vi "1_Object_Detection(Train).vi"() -> ()   [LabVIEW 2020]
doc: "This example demonstrates the usage of Deep Learning Toolkit for solving Object Detection problem with Convolutional Neural Network (CNN).\nDataset: Synthetic. Please generate the dataset with \"Dataset_Generation.vi\" in the project.\nRequirements: \n1. Deep Learning Toolkit for LabVIEW.\n2. Vision Development Module."
uses:
  <vilib>/Ngene/Deep Learning Toolkit/Toolkit/NN_Train/Controls/NN_Train_Session_Data.ctl
  <vilib>/Ngene/Deep Learning Toolkit/Toolkit/NN_Train/Controls/NN_LR_Policy_Cfg.ctl
  <vilib>/Ngene/Deep Learning Toolkit/Toolkit/NN_Train/Controls/NN_LR_Policy_Type.ctl
  <vilib>/Ngene/Deep Learning Toolkit/Toolkit/NN_Train/Controls/NN_Train_Params.ctl
  <vilib>/Ngene/Deep Learning Toolkit/Toolkit/NN_Train/Controls/NN_Train_Optimizer.ctl
  <vilib>/Ngene/Deep Learning Toolkit/Toolkit/NN_Train/Controls/NN_Train_Data_Sampling.ctl
  <vilib>/Ngene/Deep Learning Toolkit/Toolkit/NN_Network/Controls/NN_Device.ctl
  <vilib>/Ngene/Deep Learning Toolkit/Toolkit/NN_Loss/API/Controls/NN_Loss_Stats(YOLO_v2).ctl
  <vilib>/Ngene/Deep Learning Toolkit/Toolkit/NN_Data/API/NN_Dims(C,H,W).ctl
  <vilib>/Ngene/Deep Learning Toolkit/Toolkit/NN_Layers/Layers/Input/Controls/NN_Layer_Config(Input3D).ctl
  <vilib>/Ngene/Deep Learning Toolkit/Toolkit/NN_Data/Controls/NN_Data_type.ctl
  <vilib>/Ngene/Deep Learning Toolkit/Toolkit/NN_Network/Controls/NN_Save_Before_Destroy_Options.ctl
  <vilib>/Ngene/Deep Learning Toolkit/Toolkit/NN_Loss/Controls/NN_Loss_Config_Params(YOLO_v4).ctl
  <vilib>/Ngene/Deep Learning Toolkit/Toolkit/NN_Layers/Layers/YOLO_v4/delta_IOU/Controls/IOU_LOSS.ctl
  <vilib>/Ngene/Deep Learning Toolkit/Toolkit/NN_Layers/Layers/Conv2D/Controls/NN_Layer_Config(Conv2D).ctl
  <vilib>/Ngene/Deep Learning Toolkit/Toolkit/NN_Layers/Layers/Conv2D/Controls/NN_Layer_Params(Conv2D).ctl
  <vilib>/Ngene/Deep Learning Toolkit/Toolkit/NN_Layers/Layers/Conv2D/Controls/NN_Conv2D_Padding_Type.ctl
  <vilib>/Ngene/Deep Learning Toolkit/Toolkit/NN_Layers/Layers/BatchNorm/Controls/NN_BN_Params.ctl
  <vilib>/Ngene/Deep Learning Toolkit/Toolkit/NN_Activations/Controls/NN_Activation_Type.ctl
  <vilib>/Ngene/Deep Learning Toolkit/Toolkit/NN_Layers/Controls/NN_Layer_Init_Params.ctl
  <vilib>/Ngene/Deep Learning Toolkit/Toolkit/NN_Layers/Controls/NN_Layer_Weight_Init_Type.ctl
  <vilib>/Ngene/Deep Learning Toolkit/Toolkit/NN_Layers/Layers/YOLO_v4/API/Controls/NN_Layer_Config(YOLO_v4).ctl
  <vilib>/Ngene/Deep Learning Toolkit/Toolkit/NN_Layers/Layers/YOLO_v4/Controls/NN_Layer_Params(YOLO_v4).ctl
  <vilib>/Ngene/Deep Learning Toolkit/Toolkit/NN_Layers/Layers/YOLO_v4/Controls/Box_H_W_Activation_YOLO_v4.ctl
  <vilib>/Ngene/Deep Learning Toolkit/Toolkit/NN_Layers/Layers/DropOut3D/Controls/NN_Layer_Config(DropOut3D).ctl
  94310c40-c364-43de-9d18-57e5de7a2e72.vi
  <vilib>/Ngene/Deep Learning Toolkit/Toolkit/Utils/Vision/Coords_Rect2PolyLine.vi
  <vilib>/Ngene/Deep Learning Toolkit/Toolkit/NN_Layers/Layers/Input/NN_Layer_Create(Input3D).vi
  <vilib>/Ngene/Deep Learning Toolkit/Toolkit/NN_Layers/Layers/Conv2D/NN_Layer_Create(Conv2D).vi
  <vilib>/Ngene/Deep Learning Toolkit/Toolkit/NN_Layers/Layers/DropOut3D/NN_Layer_Create(DropOut3D).vi
  <vilib>/Ngene/Deep Learning Toolkit/Toolkit/NN_Layers/Layers/YOLO_v4/NN_Layer_Create(YOLO_v4).vi
  <vilib>/Ngene/Deep Learning Toolkit/Toolkit/NN_Train/Loss_Functions/NN_Set_Loss(YOLO_v4).vi
  <vilib>/Ngene/Deep Learning Toolkit/Toolkit/NN_Data/subVIs/Dataset/NN_Variant_to_DVR/4D/NN_Data_Variant_to_DVR(4D_SGL).vi
  <vilib>/Ngene/Deep Learning Toolkit/Toolkit/NN_Data/subVIs/Get_Data_Vals/4D/NN_Data_Get_ValByRef(4D_SGL_idx).vi
  <vilib>/Ngene/Deep Learning Toolkit/Toolkit/NN_Network/API/NN_Set_Input/3D/NN_Set_Input(3D_SGL_idx).vi
  <vilib>/Ngene/Deep Learning Toolkit/Toolkit/NN_Network/subVIs/NN_Predict/NN_Predict(In3D_OutBBox).vi
  <vilib>/Ngene/Deep Learning Toolkit/Toolkit/NN_Train/Eval_Loss/NN_Eval_Test_Error_Loss/NN_Eval(In3D_OutBBox).vi
  <vilib>/Ngene/Deep Learning Toolkit/Toolkit/NN_Data/subVIs/Dataset_Destroy/NN_Datasets_All_Destroy(In3D_OutBBox).vi
  <vilib>/Ngene/Deep Learning Toolkit/Toolkit/Deep_Learning_Toolkit_by_Ngene.lvlib
panel:
  in  "Eval Every N Epochs":i32=5
  out "Test.Dataset_Size":i32=74
  out "Train.Dataset_Size":i32=1224
  out "Dims_In":T1={"C"=3, "H"=320, "W"=568}
  in  "Test Dataset (Annotations)":path=path "D:/Ngene/GitHub/deepltk_examples/3_Image_Processing/33_Object_Detection/Dataset/0_Orig/Test/Annotations"
  in  "Test Dataset (Images)":path=path "D:/Ngene/GitHub/deepltk_examples/3_Image_Processing/33_Object_Detection/Dataset/0_Orig/Test/Images"
  in  "Train Dataset (Annotations)":path=path "D:/Ngene/GitHub/deepltk_examples/3_Image_Processing/33_Object_Detection/Dataset/1_Aug(4x)/Train/Annotations"
  out "Train Speed (img/s)":dbl=167.44125689875221 format="%#_2p"
  out "Session Data":T2={"Epochs"=18.130718, "Tot_Iter"=1387, "LR"=0.005, "LR_iter"=1388}
  in  "Stop":bool
  in  "LR Update Policy":T3={"Policy_Type"=enum."Step", "LR0"=0.01, "k"=15.0, "WarmUp_Policy"=enum."Ramp", "WarmUp_Iter"=1000, "WarmUp_Ratio"=10.0} {"WarmUp_Ratio" min=1; "WarmUp_Iter" min=1; "LR0" format="%.7f"}
  out "Train Speed (s/iter)":dbl=0.09555589999945369 format="%#_2p"
  in  "Train_Params":T5={"Optimizer"=enum."Adam", "Beta_1"=0.9, "Beta_2"=0.999, "Weight Decay(L1)"=4e-07, "Weight Decay(L2)"=4e-07, "Data_Sampling"=enum."Random"}
  out "Time_Elapsed":dbl=141.26338669999677 format="%<%H:%M:%S>t"
  in  "Working Dir":path=path "D:/working"
  in  "NN_Device":T8=enum."GPU"
  in  "Train Dataset (Images)":path=path "D:/Ngene/GitHub/deepltk_examples/3_Image_Processing/33_Object_Detection/Dataset/1_Aug(4x)/Train/Images"
  out "Loss_Stats":T9={"Avg_Recall"=0.994248, "Avg_Class"=0.99027264, "Avg_Obj"=0.814741, "Avg_IOU"=0.83733565, "Avg_NoObj"=0.014255692, "Count"=267, "Loss"=6.247297} {"Loss" format="%.5f"; "Count" format="%.5f"; "Avg_NoObj" format="%.5f"; "Avg_IOU" format="%.5f"; "Avg_Obj" format="%.5f"; "Avg_Class" format="%.5f"; "Avg_Recall" format="%.5f"}
  out "Loss_Stats_Graph":T10(graph)={"Avg_recall"=0.994248, "Avg_cat"=0.814741, "Avg_obj"=0.83733565, "Avg_iou"=0.014255692, "Avg_NoObj"=6.247297, "Count"=0.80606145, "Loss"=0.98615247}
  out "Prediction":T11(plugin-control)
  in  "IOU_Thresh(NMS)":sgl=0.42
  in  "Confidence_Thresh":sgl=0.49999997
  in  "Display?":bool
  in  "Evaluate":bool
  out "Mean_IoU":sgl=0.80606145 format="%#_4g"
  out "mAP":sgl=0.98615247 format="%#_4g"
  in  "Select Sample":i32=14 min=0 max=73 step=1
  # "4. In order to be able to observe detection results on a specific sample in a dataset set \"Display?\" to True and select sample with help of \"Select Sample\" control.\n7. Change the \"Confidence_Threshold\" and  \"IOU_Thresh(NMS)\" to observe their influence on detection results.\n8. Unselect \"Display\" button to speed up the training.\n10. Press \"Evaluate\" to measure network performance on Test dataset..\n11.  Stop the training when Loss is not decreasing any more.\n12. (Optional) Change \"NN_Device\" value to \"GPU\" to compare execution speeds on GPU and CPU.\n\nMore Examples:  https://github.com/ngenehub/deepltk_examples"
  # "Overview: This example demonstrates the usage of Deep Learning Toolkit for solving Object Detection problem with Convolutional Neural Network (YOLO v4).\nRequirements: \n1. Deep Learning Toolkit for LabVIEW.\n2. Vision Development Module.\nInstructions:\n1. Provide paths to Training and Test datasets at \"Train Dataset (Images)\", \"Train Dataset (Annotations)\", \"Test Dataset (Images)\", and \"Test Dataset (Annotations)\". \n2. Set appropriate path at \"Working Dir\" control where the results of the training will be stored.\n3. Run the VI with current configuration of parameters and observe the training process."
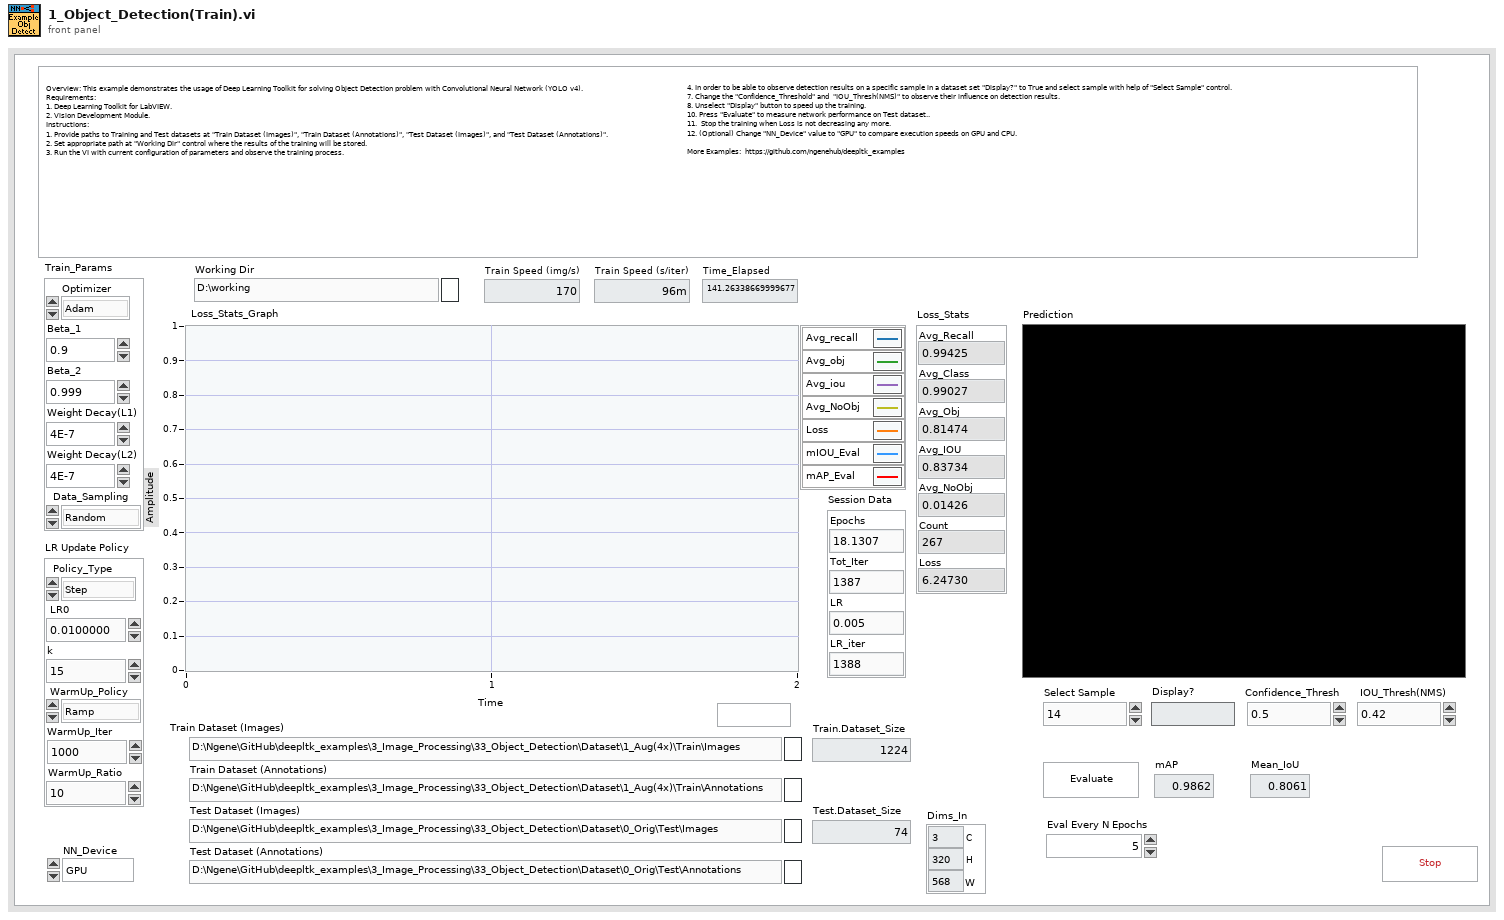
[diagram p1: front panel]
types:
  T1 = typedef "Deep_Learning_Toolkit_by_Ngene.lvlib/NN_Dims(C,H,W).ctl" = cluster{"C":i32, "H":i32, "W":i32}
  T2 = typedef "Deep_Learning_Toolkit_by_Ngene.lvlib/NN_Train_Session_Data.ctl" = cluster{"Epochs":sgl, "Tot_Iter":i32, "LR":sgl, "LR_iter":i32}
  T3 = typedef "Deep_Learning_Toolkit_by_Ngene.lvlib/NN_LR_Policy_Cfg.ctl" = cluster{"Policy_Type":T4, "LR0":dbl, "k":sgl, "WarmUp_Policy":enum16{"Step", "Ramp"}, "WarmUp_Iter":i32, "WarmUp_Ratio":sgl}
  T4 = typedef "Deep_Learning_Toolkit_by_Ngene.lvlib/NN_LR_Policy_Type.ctl" = enum16{"Manual", "Step", "Exp", "1/t"}
  T5 = typedef "Deep_Learning_Toolkit_by_Ngene.lvlib/NN_Train_Params.ctl" = cluster{"Optimizer":T6, "Beta_1":sgl, "Beta_2":sgl, "Weight Decay(L1)":sgl, "Weight Decay(L2)":sgl, "Data_Sampling":T7}
  T6 = typedef "Deep_Learning_Toolkit_by_Ngene.lvlib/NN_Train_Optimizer.ctl" = enum16{"SGD", "Adam", "Adagrad", "Adadelta", "RMSProp", "Nesterov"}
  T7 = typedef "Deep_Learning_Toolkit_by_Ngene.lvlib/NN_Train_Data_Sampling.ctl" = enum16{"Random", "Sequential"}
  T8 = typedef "Deep_Learning_Toolkit_by_Ngene.lvlib/NN_Device.ctl" = enum16{"CPU", "GPU"}
  T9 = typedef "Deep_Learning_Toolkit_by_Ngene.lvlib/NN_Loss_Stats(YOLO_v2).ctl" = cluster{"Avg_Recall":sgl, "Avg_Class":sgl, "Avg_Obj":sgl, "Avg_IOU":sgl, "Avg_NoObj":sgl, "Count":i32, "Loss":sgl}
  T10 = cluster{"Avg_recall":sgl, "Avg_cat":sgl, "Avg_obj":sgl, "Avg_iou":sgl, "Avg_NoObj":sgl, "Count":sgl, "Loss":sgl}
  T11 = typedef "IMAQ Image.ctl" = refnum<image>
  T12 = typedef "Deep_Learning_Toolkit_by_Ngene.lvlib/NN_Layer_Config(DropOut3D).ctl" = cluster{"Name":string, "Probability":sgl}
  T13 = typedef "Deep_Learning_Toolkit_by_Ngene.lvlib/NN_Layer_Config(YOLO_v4).ctl" = cluster{"Name":string, "YOLO_v4_Params":T14, "Custom_Params":string}
  T14 = typedef "Deep_Learning_Toolkit_by_Ngene.lvlib/NN_Layer_Params(YOLO_v4).ctl" = cluster{"classes":i32, "anchors":sgl[][], "Box_H_W_Activation":T15, "Box_H_W_Scale":sgl, "Box_X_Y_Scale":sgl}
  T15 = typedef "Deep_Learning_Toolkit_by_Ngene.lvlib/Box_H_W_Activation_YOLO_v4.ctl" = enum16{"Exponent", "Sigmoid"}
  T16 = typedef "Deep_Learning_Toolkit_by_Ngene.lvlib/NN_Layer_Config(Conv2D).ctl" = cluster{"Name":string, "Conv_Params":T17, "BN?":bool, "BN_Params":T19, "Activation":T20, "Has Bias?":bool, "Init_Params":T21, "Custom_Params":string}
  T17 = typedef "Deep_Learning_Toolkit_by_Ngene.lvlib/NN_Layer_Params(Conv2D).ctl" = cluster{"Filters":i32, "Kernel_Size":i32, "Stride":i32, "Pad_Type":T18, "Pad_Size":i32}
  T18 = typedef "Deep_Learning_Toolkit_by_Ngene.lvlib/NN_Conv2D_Padding_Type.ctl" = enum16{"Pad_Size", "Valid", "Same"}
  T19 = typedef "Deep_Learning_Toolkit_by_Ngene.lvlib/NN_BN_Params.ctl" = cluster{"epsilon":sgl, "momentum":sgl}
  T20 = typedef "Deep_Learning_Toolkit_by_Ngene.lvlib/NN_Activation_Type.ctl" = enum16{"Sigmoid", "ReLU", "LReLU", "ReLU6", "tanh", "Swish", "Mish", "None"}
  T21 = typedef "Deep_Learning_Toolkit_by_Ngene.lvlib/NN_Layer_Init_Params.ctl" = cluster{"Init_Type":T22, "Value":sgl}
  T22 = typedef "Deep_Learning_Toolkit_by_Ngene.lvlib/NN_Layer_Weight_Init_Type.ctl" = enum16{"Const", "Uniform", "Gaussian", "Xavier"}
  T23 = typedef "Deep_Learning_Toolkit_by_Ngene.lvlib/NN_Loss_Config_Params(YOLO_v4).ctl" = cluster{"noobject_conf_thresh ":sgl, "object_scale":sgl, "class_scale":sgl, "coord_scale":sgl, "noobject_scale":sgl, "obj_to_IOU_power":sgl, "IOU_loss":T24}
  T24 = typedef "Deep_Learning_Toolkit_by_Ngene.lvlib/IOU_LOSS.ctl" = enum16{"MSE", "IOU", "GIOU", "DIOU", "CIOU"}
  T25 = typedef "Image Type" = u32
  T26 = typedef "Deep_Learning_Toolkit_by_Ngene.lvlib/NN_Save_Before_Destroy_Options.ctl" = cluster{"CFG?":bool, "Weights?":bool, "Render?":bool}
  T27 = typedef "Deep_Learning_Toolkit_by_Ngene.lvlib/NN_Layer_Config(Input3D).ctl" = cluster{"Name":string, "Dims":T1, "Data_Type":T28, "Shifts":sgl[], "Scales":sgl[]}
  T28 = typedef "Deep_Learning_Toolkit_by_Ngene.lvlib/NN_Data_type.ctl" = enum16{"I8", "U8", "I16", "U16", "U32 ARGB", "SGL"}
  T29 = typedef "Deep_Learning_Toolkit_by_Ngene.lvlib/NN_DataSets_All(In3D_OutBBox).ctl" = cluster{"Train":T30, "Validation":T30, "Test":T30}
  T30 = typedef "Deep_Learning_Toolkit_by_Ngene.lvlib/NN_DataSet(In3D_OutBBox).ctl" = cluster{"Inputs Ref.":variant, "Dataset_Size":i32, "Dims_In":T1, "Outputs Refs":T31, "No of Classes ":i32, "Labels":string[], "File Paths":path[]}
  T31 = typedef "Deep_Learning_Toolkit_by_Ngene.lvlib/NN_Data_ref(1D_BBox).ctl" = refnum<data-value>
  T32 = typedef "Deep_Learning_Toolkit_by_Ngene.lvlib/NN.ctl" = cluster{"Name":string, "No of Layers":i32, "mBatch":i32, "Layers":T33[], "Dimty":T34, "Dims_In":T1, "Dims_Out":T1, "Working_Dir":path, "Train?":bool, "Train_Params":T5, "LR_Update_Policy":T3, "Session Data":T2, "Ground_truth":T35, "NNg_hdls":T36, "NN_Device":T8, "GPU Id":i32, "Labels":string[], "Receptive Field":T37[], "Loss_Type":T38, "Loss_Cfg_Prms":variant, "NNG_WS":T39}
  T33 = typedef "Deep_Learning_Toolkit_by_Ngene.lvlib/NN_Layer_ref.ctl" = refnum<data-value>
  T34 = typedef "Deep_Learning_Toolkit_by_Ngene.lvlib/NN_In_Out_Dim-ty.ctl" = enum8{"In1D_Out1D", "In3D_Out1D", "In3D_Out3D", "In3D_OutBBox"}
  T35 = typedef "Deep_Learning_Toolkit_by_Ngene.lvlib/NN_Ground_truth.ctl" = cluster{"Y":variant}
  T36 = typedef "Deep_Learning_Toolkit_by_Ngene.lvlib/nng_cuda_handles.ctl" = cluster{"cudnn":u64, "cublas":u64, "stream":u64, "curand":u64}
  T37 = typedef "Deep_Learning_Toolkit_by_Ngene.lvlib/NN_Dims(V,H).ctl" = cluster{"V":i32, "H":i32}
  T38 = typedef "Deep_Learning_Toolkit_by_Ngene.lvlib/NN_Loss_Type.ctl" = enum16{"None", "MSE", "CrossEntropy", "YOLO_v2", "YOLO_v4"}
  T39 = typedef "Deep_Learning_Toolkit_by_Ngene.lvlib/NNG_WS.ctl" = cluster{"NNG_WS_Mem":T40, "Max_WS_Size":i64}
  T40 = typedef "Deep_Learning_Toolkit_by_Ngene.lvlib/NNg_WS_Mem_DVR.ctl" = refnum<data-value>
  T41 = typedef "Deep_Learning_Toolkit_by_Ngene.lvlib/NN_Data_ref(4D_SGL).ctl" = refnum<data-value>
  T42 = typedef "Deep_Learning_Toolkit_by_Ngene.lvlib/NN_Layer.ctl" = cluster{"Name":string, "Layer_Data":variant, "Layer_Type":T43, "Dims_In":T1, "Layers_In":variant, "Dims_Out":T1, "Layers_Out":variant, "Metrics":T44, "GPU_Data":variant, "mBatch":i32, "NN_Device":T8, "NNg_hdls":T36, "Train?":bool, "Dimty":T45, "RecptField":T46}
  T43 = typedef "Deep_Learning_Toolkit_by_Ngene.lvlib/NN_Layer_Type.ctl" = enum16{"Input1D", "Input3D", "Conv1D", "Conv2D", "Conv2D_Adv", "MaxPool", "AvgPool", "UpSample", "DropOut3D", "ShortCut", "Concat", "SoftMax3D", "FC", "DropOut", "Softmax", "Flatten", "YOLO_v2", "YOLO_v4", "Activation", "BatchNormalization", "Unsupported"}
  T44 = typedef "Deep_Learning_Toolkit_by_Ngene.lvlib/NN_Layer_Metrics.ctl" = cluster{"Data":dbl, "Params":dbl, "Ops":dbl}
  T45 = typedef "Deep_Learning_Toolkit_by_Ngene.lvlib/NN_Layer_Dimty.ctl" = enum16{"1D", "3D"}
  T46 = typedef "Deep_Learning_Toolkit_by_Ngene.lvlib/NN_Layer_RF_State.ctl" = cluster{"Dims":T37, "J":T37}
  T47 = typedef "Deep_Learning_Toolkit_by_Ngene.lvlib/NN_BBox_Detection.ctl" = cluster{"Class":i32, "Conf Level":sgl, "BBox":T48}
  T48 = typedef "Deep_Learning_Toolkit_by_Ngene.lvlib/NN_BBox.ctl" = cluster{"x":sgl, "y":sgl, "w":sgl, "h":sgl}
  T49 = cluster{"Avg_recall":sgl, "Avg_obj":sgl, "Avg_iou":sgl, "Avg_NoObj":sgl, "Loss":sgl, "Mean_IoU":sgl, "mAP":sgl}
  T50 = typedef "Deep_Learning_Toolkit_by_Ngene.lvlib/NN_Image_Detections.ctl" = cluster{"Image Detections":T47[]}
  T51 = typedef "Deep_Learning_Toolkit_by_Ngene.lvlib/NN_Eval_Params(in3D_OutBBox).ctl" = cluster{"Precision@Max_Avg_F1_Score":sgl, "Recall@Max_Avg_F1_Score":sgl, "argmax_avgF1_Score(Conf)":sgl, "Max_Avg_F1_Score":sgl, "Max_F1_Score_Per_Class":sgl[], "F1_Score_Per_Class":sgl[][], "Avg_F1,P,R Curves":cluster{"Conf":sgl[], "F1|P|R":sgl[]}[], "mIOU":sgl, "APs@0.5":sgl[], "PR_Curves@0.5":T52, "IOUs":sgl[], "mAP@0.75":sgl, "mAP@0.5-0.95":sgl, "mAP@0.5":sgl, "Mean_PR_Curve":T53}
  T52 = typedef "Deep_Learning_Toolkit_by_Ngene.lvlib/NN_PR_Curves.ctl" = T53[]
  T53 = typedef "Deep_Learning_Toolkit_by_Ngene.lvlib/NN_PR.ctl" = cluster{"Recall":sgl[], "Precision":sgl[]}
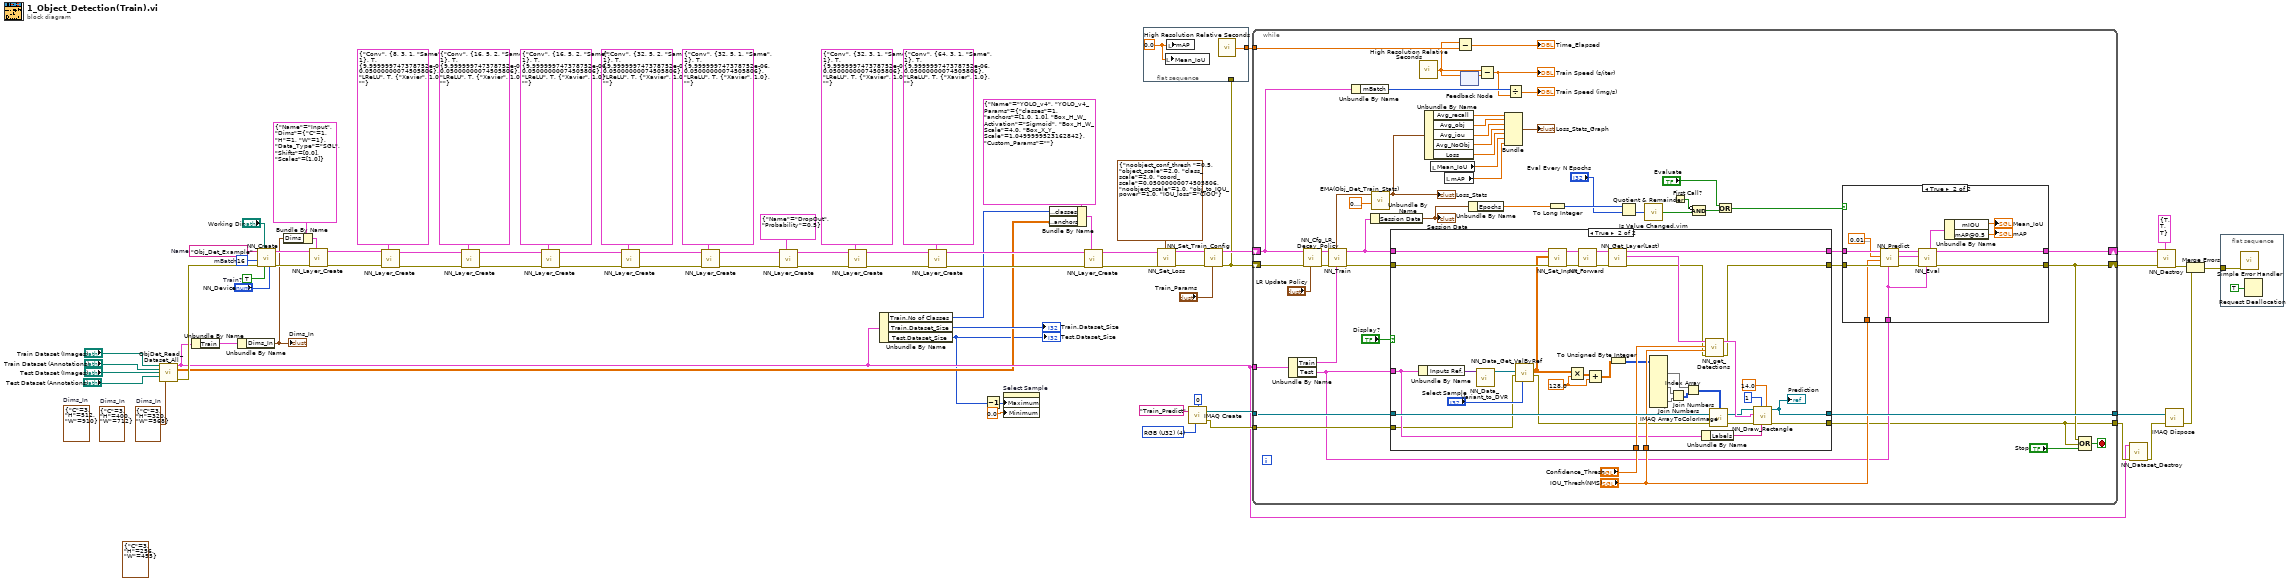
[diagram p0: block diagram]
diagram:
  (unwired) T1 {"C"=3, "H"=400, "W"=712}  # Dims_In
  w1 = T1 {"C"=3, "H"=320, "W"=568}  # Dims_In
  (unwired) T1 {"C"=3, "H"=256, "W"=455} ("Dims(C,H,W)")
  (unwired) T1 {"C"=3, "H"=512, "W"=910}  # Dims_In
  w52 = T25 4 items=["Grayscale (U8)", "Grayscale (I16)", "Grayscale (SGL)", "Complex (CSG)", "RGB (U32)", "HSL (U32)", "RGB (U64)", "Grayscale (U16)"] ("Image Type")
  w61 = TRUE  # Train?
  w67 = 16  # mBatch
  w74 = "Obj_Det_Example"  # Name
  n1 = call "ObjDet_Read_Dataset_All.vi"("Train Image Path"="Train Dataset (Images)", "Train Anno Path"="Train Dataset (Annotations)", "Test Image Path"="Test Dataset (Images)", "Test Anno Path"="Test Dataset (Annotations)", "Dims(C,H,W)"=w1) -> ("Dataset"=w33:T29, "Anchors"=w30:dbl[][], "error out"=w75:errorcluster)  [unwired: 8 in]
  n2 = Unbundle By Name(w33) -> ("Train"=w40:T30)
  n3 = Unbundle By Name(w40) -> ("Dims_In"=w34:T1)
  "Dims_In" <- w34
  n4 = call <vilib>:"NN_Create.vi"("NN_Device"="NN_Device", "Train? (false)"=w61, "Working Dir"="Working Dir", "error in (no error)"=w75, "mBatch (1)"=w67, "Name"=w74) -> ("error out"=w72:errorcluster, "NN out"=w73:T32)  [unwired: 4 in]
  n5 = Bundle By Name(cluster=T27 {"Name"="Input", "Dims"={"C"=1, "H"=1, "W"=1}, "Data_Type"=enum."SGL", "Shifts"=[0.0], "Scales"=[1.0]} ("Cluster"), "Dims"=w34) -> (w37:T27)
  n6 = call-poly <vilib>:"NN_Layer_Create.vi"("Input3D_Cfg"=w37, "error in (no error)"=w72, "NN In"=w73) -> ("error out"=w58:errorcluster, "NN out"=w41:T32)  [unwired: 6 in, 1 out]
  n7 = call-poly <vilib>:"NN_Layer_Create.vi"("Conv2D_Cfg"=T16 {"Name"="Conv", "Conv_Params"={"Filters"=8, "Kernel_Size"=3, "Stride"=1, "Pad_Type"=enum."Same", "Pad_Size"=1}, "BN?"=TRUE, "BN_Params"={"epsilon"=1e-05, "momentum"=0.05}, "Activation"=enum."LReLU", "Has Bias?"=TRUE, "Init_Params"={"Init_Type"=enum."Xavier", "Value"=1.0}, "Custom_Params"=""} ("Layer_Config_Params"), "error in (no error)"=w58, "NN in"=w41) -> ("error out"=w13:errorcluster, "NN out"=w14:T32)  [unwired: 6 in, 1 out]
  n8 = call-poly <vilib>:"NN_Layer_Create.vi"("Conv2D_Cfg"=T16 {"Name"="Conv", "Conv_Params"={"Filters"=16, "Kernel_Size"=5, "Stride"=2, "Pad_Type"=enum."Same", "Pad_Size"=1}, "BN?"=TRUE, "BN_Params"={"epsilon"=1e-05, "momentum"=0.05}, "Activation"=enum."LReLU", "Has Bias?"=TRUE, "Init_Params"={"Init_Type"=enum."Xavier", "Value"=1.0}, "Custom_Params"=""} ("Layer_Config_Params"), "error in (no error)"=w13, "NN in"=w14) -> ("error out"=w21:errorcluster, "NN out"=w22:T32)  [unwired: 6 in, 1 out]
  n9 = call-poly <vilib>:"NN_Layer_Create.vi"("Conv2D_Cfg"=T16 {"Name"="Conv", "Conv_Params"={"Filters"=16, "Kernel_Size"=5, "Stride"=2, "Pad_Type"=enum."Same", "Pad_Size"=1}, "BN?"=TRUE, "BN_Params"={"epsilon"=1e-05, "momentum"=0.05}, "Activation"=enum."LReLU", "Has Bias?"=TRUE, "Init_Params"={"Init_Type"=enum."Xavier", "Value"=1.0}, "Custom_Params"=""} ("Layer_Config_Params"), "error in (no error)"=w21, "NN in"=w22) -> ("error out"=w17:errorcluster, "NN out"=w18:T32)  [unwired: 6 in, 1 out]
  n10 = call-poly <vilib>:"NN_Layer_Create.vi"("Conv2D_Cfg"=T16 {"Name"="Conv", "Conv_Params"={"Filters"=32, "Kernel_Size"=5, "Stride"=2, "Pad_Type"=enum."Same", "Pad_Size"=1}, "BN?"=TRUE, "BN_Params"={"epsilon"=1e-05, "momentum"=0.05}, "Activation"=enum."LReLU", "Has Bias?"=TRUE, "Init_Params"={"Init_Type"=enum."Xavier", "Value"=1.0}, "Custom_Params"=""} ("Layer_Config_Params"), "error in (no error)"=w17, "NN in"=w18) -> ("error out"=w11:errorcluster, "NN out"=w12:T32)  [unwired: 6 in, 1 out]
  n11 = call-poly <vilib>:"NN_Layer_Create.vi"("Conv2D_Cfg"=T16 {"Name"="Conv", "Conv_Params"={"Filters"=32, "Kernel_Size"=5, "Stride"=1, "Pad_Type"=enum."Same", "Pad_Size"=1}, "BN?"=TRUE, "BN_Params"={"epsilon"=1e-05, "momentum"=0.05}, "Activation"=enum."LReLU", "Has Bias?"=TRUE, "Init_Params"={"Init_Type"=enum."Xavier", "Value"=1.0}, "Custom_Params"=""} ("Layer_Config_Params"), "error in (no error)"=w11, "NN in"=w12) -> ("error out"=w16:errorcluster, "NN out"=w4:T32)  [unwired: 6 in, 1 out]
  n12 = call-poly <vilib>:"NN_Layer_Create.vi"("DropOut3D_Cfg"=T12 {"Name"="DropOut", "Probability"=0.5}, "error in (no error)"=w16, "NN in"=w4) -> ("error out"=w5:errorcluster, "NN out"=w3:T32)  [unwired: 6 in, 1 out]
  n13 = call-poly <vilib>:"NN_Layer_Create.vi"("Conv2D_Cfg"=T16 {"Name"="Conv", "Conv_Params"={"Filters"=32, "Kernel_Size"=3, "Stride"=1, "Pad_Type"=enum."Same", "Pad_Size"=1}, "BN?"=TRUE, "BN_Params"={"epsilon"=1e-05, "momentum"=0.05}, "Activation"=enum."LReLU", "Has Bias?"=TRUE, "Init_Params"={"Init_Type"=enum."Xavier", "Value"=1.0}, "Custom_Params"=""} ("Layer_Config_Params"), "error in (no error)"=w5, "NN in"=w3) -> ("error out"=w24:errorcluster, "NN out"=w25:T32)  [unwired: 6 in, 1 out]
  n14 = Unbundle By Name(w33) -> ("Train.No of Classes"=w31:i32, "Train.Dataset_Size"=→"Train.Dataset_Size":i32, "Test.Dataset_Size"=w6:i32)
  "Test.Dataset_Size" <- w6
  n15 = call-poly <vilib>:"NN_Layer_Create.vi"("Conv2D_Cfg"=T16 {"Name"="Conv", "Conv_Params"={"Filters"=64, "Kernel_Size"=3, "Stride"=1, "Pad_Type"=enum."Same", "Pad_Size"=1}, "BN?"=TRUE, "BN_Params"={"epsilon"=1e-05, "momentum"=0.05}, "Activation"=enum."LReLU", "Has Bias?"=TRUE, "Init_Params"={"Init_Type"=enum."Xavier", "Value"=1.0}, "Custom_Params"=""} ("Layer_Config_Params"), "error in (no error)"=w24, "NN in"=w25) -> ("error out"=w38:errorcluster, "NN out"=w39:T32)  [unwired: 6 in, 1 out]
  n16 = Decrement(x=w6) -> (x-1=w8:i32)
  n17 = property on="Select Sample" class="DigNum (strict)"("Maximum"=w8, "Minimum"=0.0 ("Data Entry Limits:Minimum")) -> ()  [unwired: 2 in, 2 out]
  n18 = Bundle By Name(cluster=T13 {"Name"="YOLO_v4", "YOLO_v4_Params"={"classes"=1, "anchors"=[[1.0, 1.0]], "Box_H_W_Activation"=enum."Sigmoid", "Box_H_W_Scale"=4.0, "Box_X_Y_Scale"=1.05}, "Custom_Params"=""} ("YOLO_v4_Cfg"), "YOLO_v4_Params.classes"=w31, "YOLO_v4_Params.anchors"=w30) -> (w9:T13)
  n19 = call-poly <vilib>:"NN_Layer_Create.vi"("YOLO_v4_Cfg"=w9, "error in (no error)"=w38, "NN in"=w39) -> ("error out"=w53:errorcluster, "NN out"=w65:T32)  [unwired: 6 in, 1 out]
  n20 = flat-sequence {
    tunnel: [w77] -> w69
    tunnel: w62 -> [_]
    frame #0 {
      w76 = sgl 0.0 ("mAP")
      n21 = local write "Mean_IoU"(w76) -> ()
      n22 = local write "mAP"(w76) -> ()
      n23 = call <vilib>:"High Resolution Relative Seconds.vi"() -> ("relative seconds"=w77:dbl)
    }
  }
  n24 = call-poly <vilib>:"NN_Set_Loss.vi"("Loss_Config_Params(YOLO_v4)"=T23 {"noobject_conf_thresh "=0.5, "object_scale"=2.0, "class_scale"=2.0, "coord_scale"=0.05, "noobject_scale"=1.0, "obj_to_IOU_power"=1.0, "IOU_loss"=enum."CIOU"}, "error in (no error)"=w53, "NN in"=w65) -> ("error out"=w56:errorcluster, "NN out"=w57:T32)  [unwired: 7 in]
  n25 = call "IMAQ Create"("Border Size"=0, "Image Name"="Train_Predict", "Image Type"=w52) -> ("New Image"=w49:T11, "error out"=w48:errorcluster)  [unwired: 2 in]
  n26 = call <vilib>:"NN_Set_Train_Config.vi"("NN_Train_Params"="Train_Params", "error in (no error)"=w56, "NN in"=w57) -> ("error out"=w62:errorcluster, "NN out"=w63:T32)  [unwired: 7 in]
  n27 = while {
    shift-right: [w105] -> w66
    shift-left: w62 -> [w114]
    shift-right: [w79] -> w70
    shift-left: w63 -> [w115]
    tunnel: w69 -> [w123]
    tunnel: w49 -> [w111]
    tunnel: [w110] -> w47
    tunnel: w48 -> [w109]
    tunnel: [w78] -> w45
    tunnel: w33 -> [w101]
    stop <- w126 stop-if-true
    n28 = Unbundle By Name(w101) -> ("Train"=w99:T30, "Test"=w98:T30)
    n29 = call <vilib>:"NN_Cfg_LR_Decay_Policy.vi"("LR_Decay_Params"="LR Update Policy", "error in (no error)"=w114, "NN in"=w115) -> ("error out"=w124:errorcluster, "NN out"=w127:T32)  [unwired: 7 in]
    n30 = call <vilib>:"NN_Train.vi"("Train Dataset"=w99, "error in (no error)"=w124, "NN in"=w127) -> ("error out"=w112:errorcluster, "NN out"=w113:T32, "Det_Train_Stats"=w125:T9)  [unwired: 3 in, 3 out]
    n31 = Unbundle By Name(w115) -> ("mBatch"=w120:i32)
    n32 = Unbundle By Name(w113) -> ("Session Data"=w97:T2)
    "Session Data" <- w97
    n33 = call "EMA(Obj_Det_Train_Stats).vi"("Exp_Avg"=sgl 0.9, "Det_Train_Stats"=w125) -> ("Cluster"=w90:T10)  [unwired: 9 in]
    "Loss_Stats" <- w90
    n34 = case shown="True" "Display?" {
      tunnel: w113 -> [w145 w167]
      tunnel: w112 -> [w144 w169]
      tunnel: w111 -> [w147 w184]
      tunnel: [w147 w183] -> w110
      tunnel: w109 -> [w146 w160]
      tunnel: [w146 w182] -> w78
      tunnel: [w144 w151] -> w106
      tunnel: [w145 w180] -> w107
      tunnel: "Confidence_Thresh" -> [_ w173]
      tunnel: "IOU_Thresh(NMS)" -> [_ w172]
      tunnel: w98 -> [_ w164]
      frame False {
      }
      frame True {
        w174 = sgl 128.0 ("bias_match")
        n35 = Unbundle By Name(w164) -> ("Inputs Ref."=w161:variant)
        n36 = call-poly <vilib>:"NN_Data_Variant_to_DVR.vi"("Inputs Ref."=w161) -> ("DVR(4D_SGL)"=w150:T41)  [unwired: 9 in, 1 out]
        n37 = call-poly <vilib>:"NN_Data_Get_ValByRef.vi"("index (vol)"="Select Sample", "error in (no error)"=w160, "DVR(4D_SGL)"=w150) -> ("error out"=w149:errorcluster, "Value(3D_SGL)"=w162:sgl[][][])  [unwired: 5 in]
        n38 = call-poly <vilib>:"NN_Set_Input.vi"("error in (no error)"=w169, "Data_In(3D_SGL)"=w162, "NN in"=w167) -> ("error out"=w165:errorcluster, "NN out"=w171:T32)  [unwired: 7 in]
        n39 = Multiply(x=w162, y=w174) -> (x*y=w176:sgl[][][])
        n40 = call <vilib>:"NN_Forward.vi"("error in (no error)"=w165, "NN in"=w171) -> ("error out"=w168:errorcluster, "NN out"=w170:T32)  [unwired: 6 in, 2 out]
        n41 = Add(x=w176, y=w174) -> (x+y=w159:sgl[][][])
        n42 = call <vilib>:"NN_Get_Layer(Last).vi"("error in (no error)"=w168, "NN in"=w170) -> ("error out"=w152:errorcluster, "Last_Layer"=w181:T42, "NN out"=w180:T32)  [unwired: 6 in, 1 out]
        n43 = To Unsigned Byte Integer(number=w159) -> (unsigned 8bit integer=w158:u8[][][])
        n44 = Index Array(array=w158) -> (element #1=w154:u8[][], element #2=w155:u8[][], element #3=w156:u8[][])  [unwired: 9 in]
        n45 = Join Numbers(hi=w155, lo=w156) -> ((hi.lo)=w153:u16[][])
        n46 = Join Numbers(hi=w154, lo=w153) -> ((hi.lo)=w157:u32[][])
        n47 = Unbundle By Name(w164) -> ("Labels"=w163:string[])
        n48 = call <vilib>:"NN_get_Detections.vi"("error in"=w152, "IOU_Thrsh"=w172, "Confidence_Thrsh"=w173, "YOLO_Layer"=w181) -> ("error out"=w151:errorcluster, "Detections"=w179:T47[])  [unwired: 6 in]
        n49 = call "IMAQ ArrayToColorImage"("Image Pixels (U32)"=w157, "Image"=w184, "error in (no error)"=w149) -> ("Image Out"=w177:T11, "error out"=w148:errorcluster)  [unwired: 2 in]
        n50 = call "NN_Draw_Rectangle.vi"("font_size"=sgl 14.0, "Labels"=w163, "Border_Width"=u32 1, "error in (no error)"=w148, "Draw_Boxes"=w179, "Img in"=w177) -> ("error out"=w182:errorcluster, "Img out"=w183:T11)  [unwired: 4 in]
        "Prediction" <- w183
      }
    }
    n51 = call <vilib>:"High Resolution Relative Seconds.vi"() -> ("relative seconds"=w122:dbl)
    n52 = Unbundle By Name(w90) -> ("Avg_recall"=w89:sgl, "Avg_obj"=w88:sgl, "Avg_iou"=w87:sgl, "Avg_NoObj"=w86:sgl, "Loss"=w85:sgl)
    n53 = local read "Mean_IoU"() -> (w84:sgl)
    n54 = local read "mAP"() -> (w83:sgl)
    n55 = Subtract(x=w122, y=w123) -> (x-y=→"Time_Elapsed":dbl)
    n56 = feedback #1() -> (w128:dbl)  [unwired: 1 in]
    n57 = feedback-in #1(w122) -> ()
    n58 = Unbundle By Name(w97) -> ("Epochs"=w96:sgl)
    n59 = Subtract(x=w122, y=w128) -> (x-y=w118:dbl)
    "Train Speed (s/iter)" <- w118
    n60 = Bundle("Avg_recall"=w89, "Avg_obj"=w88, "Avg_iou"=w87, "Avg_NoObj"=w86, "Loss"=w85, "Mean_IoU"=w84, "mAP"=w83) -> (→"Loss_Stats_Graph":T49)  [unwired: 1 in]
    n61 = Divide(x=w120, y=w118) -> (x/y=→"Train Speed (img/s)":dbl)
    n62 = To Long Integer(number=w96) -> (32bit integer=w95:i32)
    n63 = Quotient & Remainder(x=w95, y="Eval Every N Epochs") -> (floor(x/y)=w92:i32)  [unwired: 1 out]
    n64 = call "Is Value Changed.vim"("value"=w92) -> ("changed or first call?"=w91:bool)
    n65 = First Call?() -> (First Call?: T/F=w80:bool)
    n66 = Compound Arithmetic op=AND(invert w80, w91) -> (w81:bool)
    n67 = Or(x="Evaluate", y=w81) -> (x .or. y?=w93:bool)
    n68 = case shown="True" w93 {
      tunnel: w107 -> [w130 w143]
      tunnel: [w130 w142] -> w79
      tunnel: w106 -> [w129 w139]
      tunnel: [w129 w141] -> w105
      tunnel: "IOU_Thresh(NMS)" -> [_ w133]
      tunnel: w98 -> [_ w132]
      frame False {
      }
      frame True {
        n69 = call-poly <vilib>:"NN_Predict.vi"("Dataset"=w132, "error in (no error)"=w139, "NMS_IOU_Thresh(0.5)"=w133, "Conf_Thresh(0.5)"=sgl 0.02, "NN in"=w143) -> ("error out"=w138:errorcluster, "Predictions"=w134:T50[], "NN out"=w140:T32)  [unwired: 4 in]
        n70 = call-poly <vilib>:"NN_Eval.vi"("Dataset"=w132, "error in"=w138, "Detections(in Dataset)"=w134, "NN in"=w140) -> ("error out"=w141:errorcluster, "NN out"=w142:T32, "NN_Eval_Params"=w137:T51)  [unwired: 5 in]
        n71 = Unbundle By Name(w137) -> ("mIOU"=→"Mean_IoU":sgl, "mAP@0.5"=→"mAP":sgl)
      }
    }
    n72 = Compound Arithmetic op=OR(w105, w78, "Stop") -> (w126:bool)
  }
  n73 = call-poly <vilib>:"NN_Dataset_Destroy.vi"("error in (no error)"=w45, "Datasets_All(In3D_OutBBox)"=w33) -> ("error out"=w44:errorcluster)  [unwired: 9 in]
  n74 = call <vilib>:"NN_Destroy.vi"("Save (T, T, T)"=T26 {"CFG?"=TRUE, "Weights?"=TRUE, "Render?"=TRUE} ("Save_Config"), "error in (no error)"=w66, "NN in"=w70) -> ("error out"=w71:errorcluster)  [unwired: 7 in, 1 out]
  n75 = call "IMAQ Dispose"("Image"=w47, "error in (no error)"=w44) -> ("error out"=w42:errorcluster)  [unwired: 4 in]
  n76 = Merge Errors(w71, w42) -> (w43:errorcluster)
  n77 = flat-sequence {
    tunnel: w43 -> [w186]
    frame #0 {
      n78 = call <vilib>:"Simple Error Handler.vi"("error in (no error)"=w186) -> ()  [unwired: 4 in, 5 out]
      n79 = Request Deallocation(TRUE ("flag")) -> ()
    }
  }
